vi "fix nivs dependency failboat.vi"(8 "error in":errorcluster, 11 "Device Item Ref in":T1 format="%.0x") -> (0 "error out":errorcluster)   [LabVIEW 2026, in "Nominal Core Streaming System Explorer.lvlib"]
uses:
  Nominal Core Streaming System Explorer.lvlib
  <vilib>/NI VeriStand/Custom Device API/Custom Device Item Ref.ctl
  <vilib>/NI VeriStand/Custom Device API/Custom Device File Dependency.ctl
  <vilib>/NI VeriStand/Custom Device API/Path Specification.ctl
  <vilib>/NI VeriStand/Custom Device API/Path Type.ctl
  <vilib>/NI VeriStand/Custom Device API/Custom Device Supported Target.ctl
  <vilib>/NI VeriStand/Custom Device API/Custom Device API.lvlib
  <vilib>/Utility/SystemLogging/NI_SystemLogging.lvlib
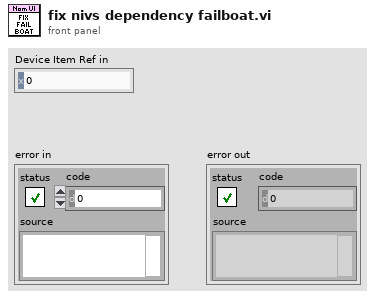
[diagram p1: front panel]
types:
  T1 = typedef "Custom Device API.lvlib/Custom Device Item Ref.ctl" = u64
  T2 = typedef "Custom Device API.lvlib/Custom Device Supported Target.ctl" = enum16{"All", "PharLap", "VxWorks", "Windows", "Linux_32_ARM", "Linux_x64", "PharLap & Windows", "PharLap & VxWorks", "VxWorks & Windows"}
  T3 = typedef "Custom Device API.lvlib/Path Type.ctl" = enum16{"Absolute", "To Base", "To Common Data Dir", "To Application Data Dir"}
  T4 = typedef "Custom Device API.lvlib/Custom Device File Dependency.ctl" = cluster{"Source":T5, "RT Destination":path, "ForceDownload?":bool, "SupportedTarget":T2, "Version":string}
  T5 = typedef "Custom Device API.lvlib/Path Specification.ctl" = cluster{"Path":path, "Type":T3}
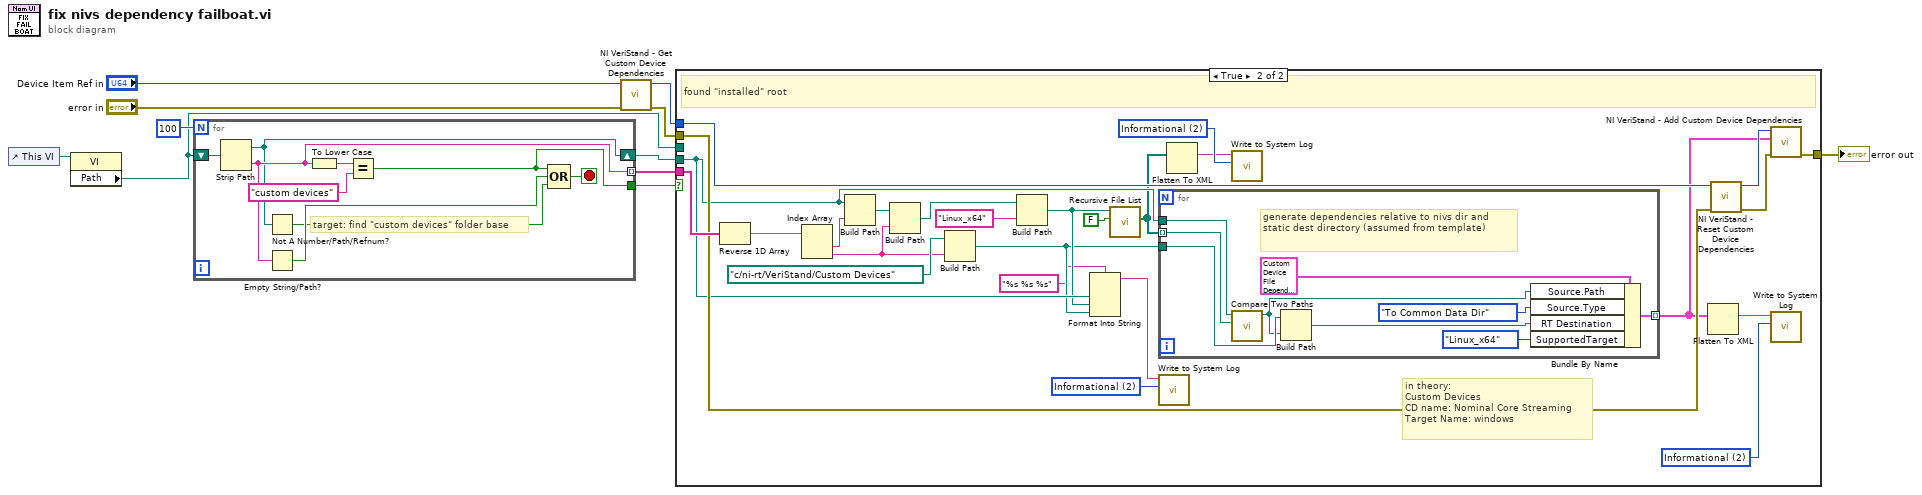
[diagram p0: block diagram]
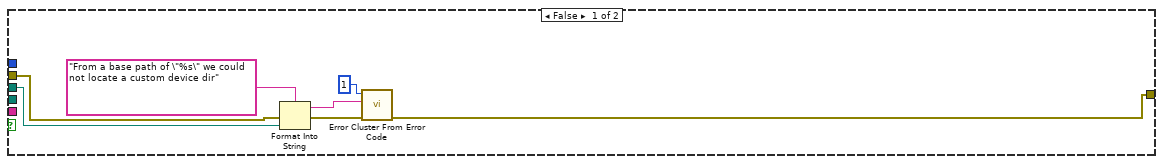
[diagram p2: hidden frame]
diagram:
  n1 = control-ref of="This VI"() -> (w9:refnum<vi>)
  n2 = property class="VI"(reference=w9) -> ("Path"=w2:path)  [unwired: 1 in, 2 out]
  n3 = for {
    N: 100 -> [_]
    shift-right: [w13] -> w6
    shift-left: w2 -> [w20]
    tunnel: [w14] -> w5 mode=indexing
    tunnel: [w17] -> w7
    stop <- w16 stop-if-true
    # "target: find \"custom devices\" folder base"
    n4 = Strip Path(path=w20) -> (stripped path=w13:path, name=w14:string)
    n5 = Not A Number/Path/Refnum?(number/path/refnum=w13) -> (NaN/Path/Refnum?=w12:bool)
    n6 = Empty String/Path?(string/path=w14) -> (empty?=w15:bool)
    n7 = To Lower Case(string=w14) -> (all lower case string=w19:string)
    n8 = Equal?(x=w19, y="custom devices") -> (x = y?=w17:bool)
    n9 = Compound Arithmetic op=OR(w17, w15, w12) -> (w16:bool)
  }
  n10 = call <vilib>:"NI VeriStand - Get Custom Device Dependencies.vi"("error in (no error)"="error in", "Device Ref in"="Device Item Ref in") -> ("error out"=w4:errorcluster, "Device Ref out"=w1:T1)  [unwired: 7 in, 1 out]
  n11 = case shown="True" w7 {
    tunnel: w6 -> [_ w36]
    tunnel: w5 -> [_ w53]
    tunnel: w4 -> [w27 w44]
    tunnel: [w26 w40] -> w3
    tunnel: w2 -> [w22 _]
    tunnel: w1 -> [_ w43]
    frame False {
      n12 = Format Into String(format string="From a base path of \"%s\" we could not locate a custom device dir", error in=w27, w22) -> (resulting string=w23:string, error out=w24:errorcluster)  [unwired: 1 in]
      n13 = call <vilib>:"Error Cluster From Error Code.vi"("error in (no error)"=w24, "error message (\"\")"=w23, "error code (0)"=1) -> ("error out"=w26:errorcluster)  [unwired: 6 in]
    }
    frame True {
      w30 = 2 items=["Error", "Warning", "Informational"] ("severity")
      w32 = 2 items=["Error", "Warning", "Informational"] ("severity")
      w37 = 2 items=["Error", "Warning", "Informational"] ("severity")
      # "in theory:\nCustom Devices\nCD name: Nominal Core Streaming\nTarget Name: windows"
      # "found \"installed\" root"
      n14 = Reverse 1D Array(array=w53) -> (reversed array=w52:string[])
      n15 = Index Array(array=w52) -> (element #1=w50:string, element #2=w45:string)  [unwired: 2 in]
      n16 = Build Path(base path=w36, name or relative path=w50) -> (appended path=w51:path)
      n17 = Build Path(base path=w51, name or relative path=w45) -> (appended path=w49:path)
      n18 = Build Path(base path=path "c:/ni-rt/VeriStand/Custom Devices", name or relative path=w45) -> (appended path=w34:path)
      n19 = Build Path(base path=w49, name or relative path="Linux_x64") -> (appended path=w35:path)
      n20 = Format Into String(format string="%s %s %s", w36, w35, w34) -> (resulting string=w29:string)  [unwired: 2 in, 1 out]
      n21 = call <vilib>:"Recursive File List.vi"("Treat LLBs as Folders?"=FALSE, "Folder Path"=w35) -> ("All Files in Dir"=w33:path[])  [unwired: 5 in, 4 out]
      n22 = for {
        tunnel: w33 -> [w61] mode=indexing
        tunnel: w36 -> [w62]
        tunnel: w34 -> [w57]
        tunnel: [w54] -> w39 mode=indexing
        # "generate dependencies relative to nivs dir and static dest directory (assumed from template)"
        n23 = call <vilib>:"Compare Two Paths.vi"("Path 2"=w61, "Path 1"=w62) -> ("Relative Path from 1 to 2"=w55:path)  [unwired: 6 in, 3 out]
        n24 = Build Path(base path=w57, name or relative path=w55) -> (appended path=w56:path)
        n25 = Bundle By Name(cluster=T4 {"Source"={"Path"=path "", "Type"=enum."Absolute"}, "RT Destination"=path "", "ForceDownload?"=FALSE, "SupportedTarget"=enum."PharLap", "Version"=""} ("Dependency"), "Source.Path"=w55, "Source.Type"=Path_Type."To Common Data Dir", "RT Destination"=w56, "SupportedTarget"=Custom_Device_Supported_Target."Linux_x64") -> (w54:T4)
      }
      n26 = call <vilib>:"Write to System Log.vi"("severity"=w30, "message"=w29) -> ()  [unwired: 9 in, 1 out]
      n27 = Flatten To XML(6:w33) -> (2:w31:string)
      n28 = call <vilib>:"Write to System Log.vi"("severity"=w32, "message"=w31) -> ()  [unwired: 9 in, 1 out]
      n29 = Flatten To XML(6:w39) -> (2:w38:string)
      n30 = call <vilib>:"NI VeriStand - Reset Custom Device Dependencies.vi"("error in (no error)"=w44, "Device Ref in"=w43) -> ("error out"=w41:errorcluster, "Device Ref out"=w42:T1)  [unwired: 8 in]
      n31 = call <vilib>:"NI VeriStand - Add Custom Device Dependencies.vi"("error in (no error)"=w41, "Dependencies"=w39, "Device Ref in"=w42) -> ("error out"=w40:errorcluster)  [unwired: 7 in, 1 out]
      n32 = call <vilib>:"Write to System Log.vi"("severity"=w37, "message"=w38) -> ()  [unwired: 9 in, 1 out]
    }
  }
  "error out" <- w3
